vi "GetHousingImage.vi"(4 "File type":T1, 5 "Disabled":bool, 6 "Background Color":u32(colorbox), 7 "image directory":path, 8 "error in":errorcluster, 11 "Knob in":refnum<class "Knob.lvclass">) -> (0 "error out":errorcluster, 3 "Knob out":refnum<class "Knob.lvclass">)   [LabVIEW 2014, in "Raspberry Pi Compatible Compiler for LabVIEW.lvlib" / "Knob.lvclass"]
uses:
  Knob.lvclass
  Control/ImageTypes.ctl
  <vilib>/Utility/miscctls.llb/LVForegroundBackgroundColorsTypeDef.ctl
  Raspberry Pi Compatible Compiler for LabVIEW.lvlib
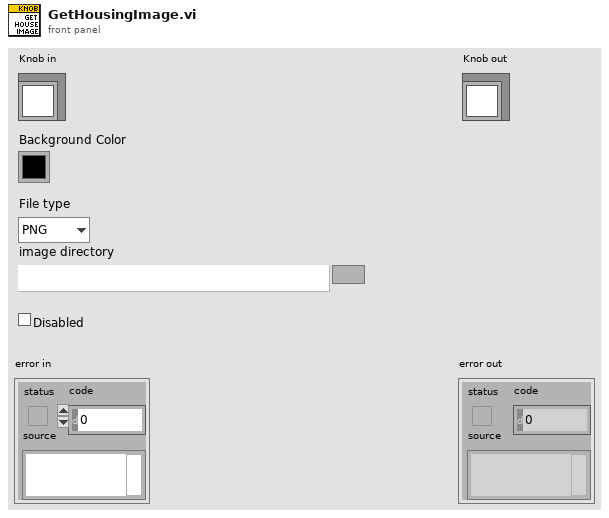
[diagram p1: front panel]
types:
  T1 = typedef "Raspberry Pi Compatible Compiler for LabVIEW.lvlib/ImageTypes.ctl" = enum16{"PNG", "JPEG", "BMP"}
  T2 = enum8{"Enabled", "Disabled", "Disabled and Grayed Out"}
  T3 = typedef "LVForegroundBackgroundColorsTypeDef.ctl" = cluster{"Foreground Color":u32, "Background Color":u32}
  T4 = typedef "imagedata.ctl" = cluster{"image type":i32, "image depth":i32, "image":u8[], "mask":u8[], "colors":u32[], "Rectangle":cluster{"left":i16, "top":i16, "right":i16, "bottom":i16}}
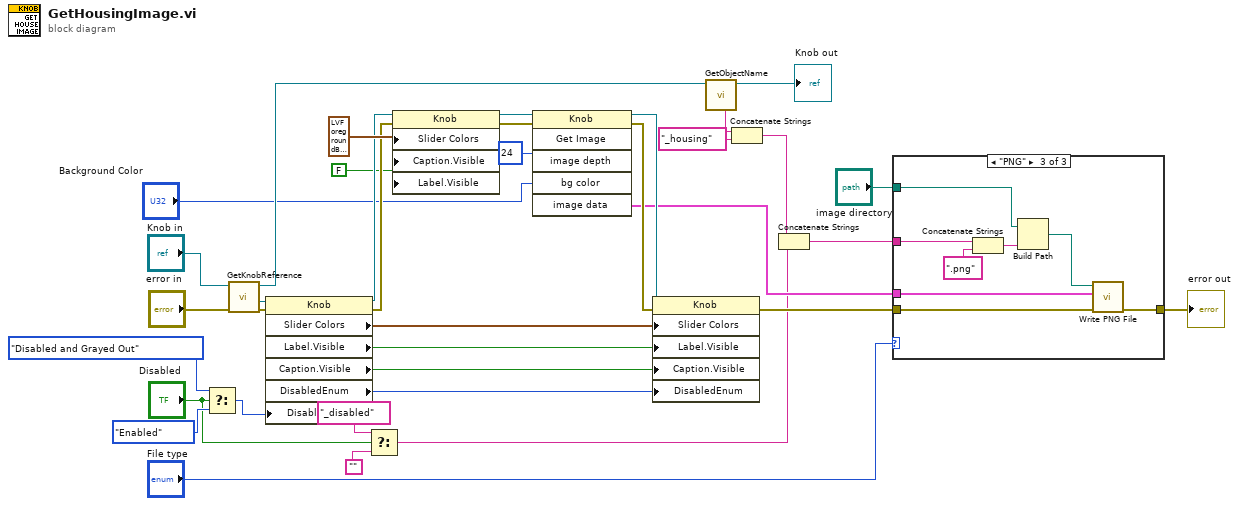
[diagram p0: block diagram]
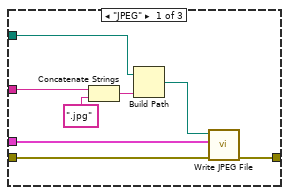
[diagram p2: hidden frame]
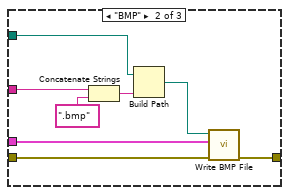
[diagram p3: hidden frame]
diagram:
  w11 = FALSE ("Caption.Visible")
  n1 = Select(t=T2."Disabled and Grayed Out" ("Disabled"), s="Disabled", f=T2."Enabled") -> (s? t:f=w7:T2)
  n2 = call "GetKnobReference.vi"("error in"="error in", "Knob in"="Knob in") -> ("error out"=w27:errorcluster, "knob reference"=w26:refnum<vi>, "Knob out"=w20:refnum<class "Knob.lvclass">)  [unwired: 7 in]
  n3 = property on="Property Node" class="Knob"(reference=w26, error in=w27, "DisabledEnum"=w7) -> (reference out=w33:refnum<vi>, error out=w34:errorcluster, "Slider Colors"=w36:T3, "Label.Visible"=w14:bool, "Caption.Visible"=w13:bool, "DisabledEnum"=w10:T2)
  n4 = Select(t="_disabled", s="Disabled", f="") -> (s? t:f=w1:string)
  n5 = property on="Property Node" class="Knob"(reference=w33, error in=w34, "Slider Colors"=T3 {"Foreground Color"=16777216, "Background Color"=16777216}, "Caption.Visible"=w11, "Label.Visible"=w11) -> (reference out=w31:refnum<vi>, error out=w30:errorcluster)
  n6 = invoke class="Knob" method="Get Image"(reference=w31, error in=w30, "image depth"=24 ("Image Depth"), "bg color"="Background Color") -> (reference out=w29:refnum<vi>, error out=w28:errorcluster, "image data"=w22:T4)  [unwired: 2 in, 3 out]
  n7 = property on="Property Node" class="Knob"(reference=w29, error in=w28, "Slider Colors"=w36, "Label.Visible"=w14, "Caption.Visible"=w13, "DisabledEnum"=w10) -> (error out=w23:errorcluster)  [unwired: 1 out]
  n8 = call-dynamic "GetObjectName.vi"("GObject in"=w20) -> ("GObject out"=→"Knob out":refnum<class "Knob.lvclass">, "Name"=w18:string)  [unwired: 6 in, 1 out]
  n9 = Concatenate Strings(w18, "_housing" ("string")) -> (w6:string)
  n10 = Concatenate Strings(w6, w1) -> (w5:string)
  n11 = case shown="\"PNG\"" "File type" {
    tunnel: w22 -> [w44 w52 w60]
    tunnel: [w43 w51 w59] -> w15
    tunnel: w23 -> [w42 w50 w58]
    tunnel: w5 -> [w41 w49 w57]
    tunnel: "image directory" -> [w37 w45 w53]
    frame "JPEG" {
      n12 = Concatenate Strings(w41, ".jpg" ("string")) -> (w39:string)
      n13 = Build Path(base path=w37, name or relative path=w39) -> (appended path=w38:path)
      n14 = call <vilib>:"Write JPEG File.vi"("error in (no error)"=w42, "image data"=w44, "path to JPEG file"=w38) -> ("error out"=w43:errorcluster)  [unwired: 7 in, 1 out]
    }
    frame "BMP" {
      n15 = Concatenate Strings(w49, ".bmp" ("string")) -> (w47:string)
      n16 = Build Path(base path=w45, name or relative path=w47) -> (appended path=w46:path)
      n17 = call <vilib>:"Write BMP File.vi"("error in (no error)"=w50, "image data"=w52, "path to BMP file"=w46) -> ("error out"=w51:errorcluster)  [unwired: 7 in, 1 out]
    }
    frame "PNG" {
      n18 = Concatenate Strings(w57, ".png" ("string")) -> (w55:string)
      n19 = Build Path(base path=w53, name or relative path=w55) -> (appended path=w54:path)
      n20 = call <vilib>:"Write PNG File.vi"("error in (no error)"=w58, "image data"=w60, "path to PNG file"=w54) -> ("error out"=w59:errorcluster)  [unwired: 7 in, 1 out]
    }
  }
  "error out" <- w15
